vi "DataPacker_CleanClose.vi"(8 "error in (no error)":errorcluster, 11 "DataPacker in":refnum<class "DataPacker.lvclass">) -> (0 "error out":errorcluster, 2 "Unsent items in queue":i32, 3 "DataPacker out":refnum<class "DataPacker.lvclass">)   [LabVIEW 2018, in "feGEM DataPacker.lvlib" / "DataPacker.lvclass"]
uses:
  DataPacker.lvclass
  DataPacker.lvclass/DataPacker.ctl
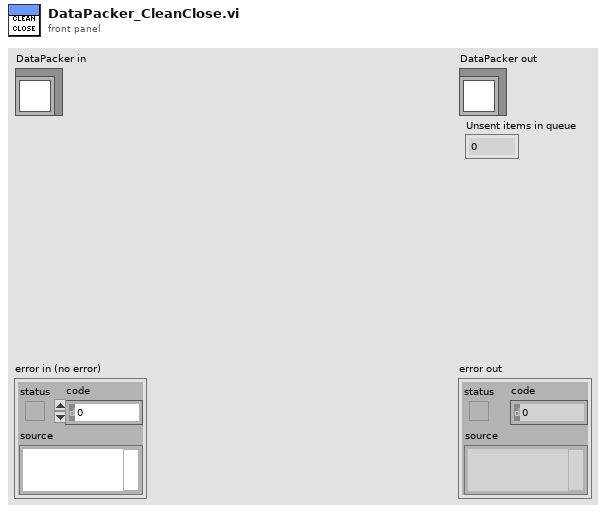
[diagram p1: front panel]
types:
  T1 = typedef "feGEM DataPacker.lvlib/GEM_BANK_CLUSTER_typedef.ctl" = cluster{"Category":string, "Variable Name":string, "Equipment description":string, "History Settings":u16, "Period to update history plots":u16, "GEM_DATA Cluster":T2}
  T2 = typedef "GEM_DATA_cluster_typedef.ctl" = cluster{"DataType":string, "Formatted Data":u8[], "data byte order (Little Endian prefered)":enum16{"big-endian, network order", "native, host order", "little-endian"}}
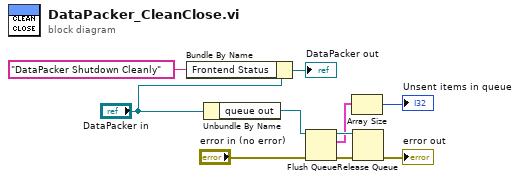
[diagram p0: block diagram]
diagram:
  n1 = Bundle By Name(cluster="DataPacker in", "Frontend Status"="DataPacker Shutdown Cleanly") -> (→"DataPacker out":refnum<class "DataPacker.lvclass">)
  n2 = Unbundle By Name("DataPacker in") -> ("queue out"=w9:refnum<queue>)
  n3 = Flush Queue(queue=w9, error in (no error)="error in (no error)") -> (queue out=w7:refnum<queue>, remaining elements=w6:T1[], error out=w3:errorcluster)
  n4 = Array Size(array=w6) -> (size(s)=→"Unsent items in queue":i32)
  n5 = Release Queue(queue=w7, error in (no error)=w3) -> (error out=→"error out":errorcluster)  [unwired: 1 in, 2 out]
